vi "MakeCommandGeneric.vi"(10 "Unique Command":string, 11 "RecievedName In":string[](array[string])) -> (0 "Handled?":bool, 1 "Unique ID":string, 2 "Generic Command":string, 3 "RecievedName Out":string[](array[string]))   [LabVIEW 2019, in "AFM_Litho_Plugin.IV.lvclass"]
uses:
  AFM_Litho_Plugin.IV.lvclass
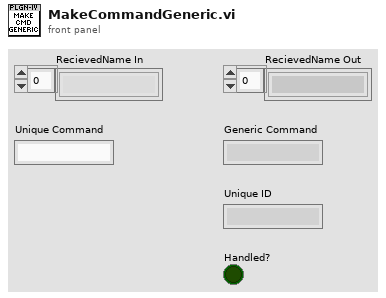
[diagram p1: front panel]
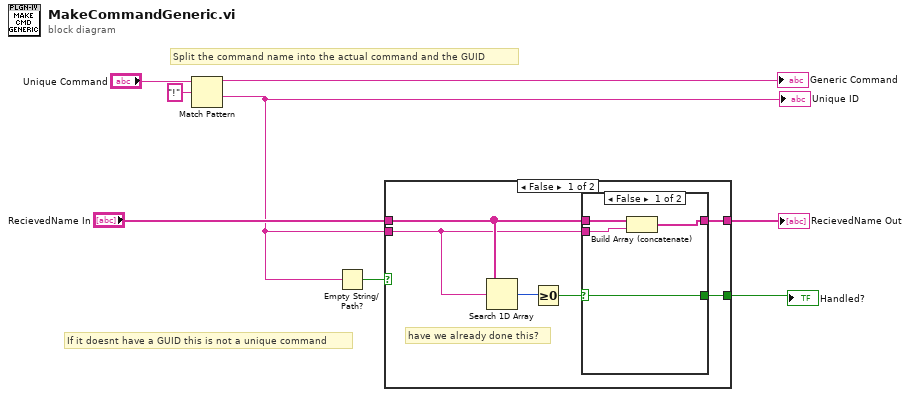
[diagram p0: block diagram]
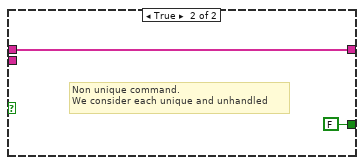
[diagram p3: hidden frame]
diagram:
  # "If it doesnt have a GUID this is not a unique command"
  # "Split the command name into the actual command and the GUID"
  n1 = Match Pattern(string="Unique Command", regular expression="!") -> (before substring=→"Generic Command":string, after substring=w2:string)  [unwired: 1 in, 2 out]
  "Unique ID" <- w2
  n2 = Empty String/Path?(string/path=w2) -> (empty?=w5:bool)
  n3 = case shown="False" w5 {
    tunnel: "RecievedName In" -> [w11 w22]
    tunnel: [w12 w22] -> w3
    tunnel: w2 -> [w10 _]
    tunnel: [w9 FALSE] -> w1
    frame False {
      # "have we already done this?"
      n4 = Search 1D Array(1D array=w11, element=w10) -> (index of element=w14:i32)  [unwired: 1 in]
      n5 = Greater Or Equal To 0?(x=w14) -> (x >= 0?=w13:bool)
      n6 = case shown="False" w13 {
        selector: w13 -> [w15 w19]
        tunnel: [w17 w20] -> w12
        tunnel: w11 -> [w18 w20]
        tunnel: w10 -> [w16 _]
        tunnel: [w15 w19] -> w9
        frame False {
          n7 = Build Array (concatenate)(w18, w16) -> (w17:string[])
        }
        frame True {
        }
      }
    }
    frame True {
      # "Non unique command.\nWe consider each unique and unhandled"
    }
  }
  "RecievedName Out" <- w3
  "Handled?" <- w1
